vi "FTW-File-SystemDirectories.vi"(1 "System Directory":i32(ring) items=["User Home"=0, "User Desktop"=1, "User Documents"=2, "User Application Data"=3, "User Preferences"=4, "User Temporary"=5, "Public Documents"=6, "Public Application Data"=7, "Public Preferences"=8, "Public Cache"=13, "System Core Libraries"=9, "System Installed Libraries"=10, "Application Files"=11, "Boot Volume Root"=12]) -> (0 "Directory":path)   [LabVIEW 2012]
panel:
  # "Inputs"
  # "Outputs"
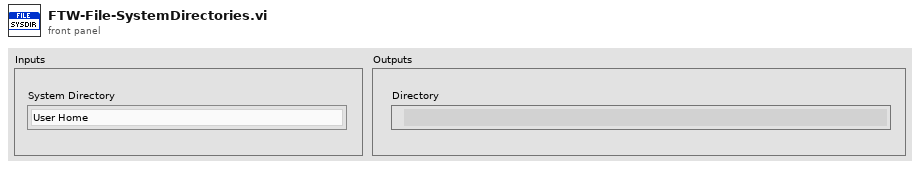
[diagram p1: front panel]
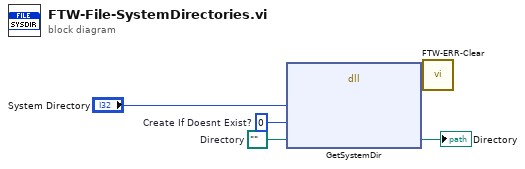
[diagram p0: block diagram]
diagram:
  w4 = path ""  # Directory
  w5 = 0  # Create If Doesnt Exist?
  n1 = dll-call lib="LabVIEW" fn="GetSystemDir"("System Directory Enum"="System Directory", "Create If Doesnt Exist"=w5, "Directory"=w4) -> (error out=w3:errorcluster, "Directory"=→"Directory":path)  [unwired: 4 in, 3 out]
  n2 = call "FTW-ERR-Clear.vi"("error to snuff"=w3) -> ()  [unwired: 1 out]
